vi "load_recipes.vi"(8 "error in (no error)":errorcluster, 11 "recipe":T2) -> (0 "error out":errorcluster, 2 "transition []":string, 3 "recipe []":T1[](array[typedef]))   [LabVIEW 2015, in "lv-recipe-machine.lvlib" / "example_01.lvlib"]
uses:
  example_01.lvlib
  _controls/recipes.ctl
  public/_controls/recipe_step.ctl
  _controls/steps_actions.ctl
  lv-recipe-machine.lvlib
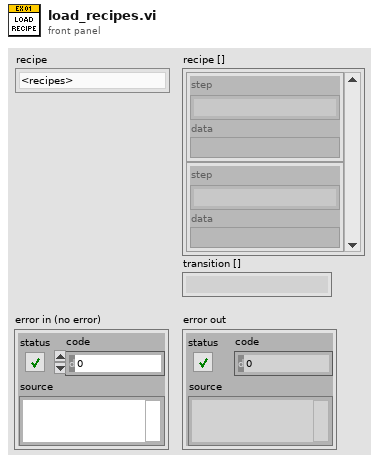
[diagram p1: front panel]
types:
  T1 = typedef "lv-recipe-machine.lvlib/recipe_step.ctl" = cluster{"step":string, "data":variant}
  T2 = typedef "lv-recipe-machine.lvlib/example_01.lvlib/recipes.ctl" = enum16{"<recipes>", "wait_random", "random_wait", "count", "comparison", "launch", "<null>"}
  T3 = typedef "lv-recipe-machine.lvlib/example_01.lvlib/steps_actions.ctl" = enum16{"<steps_actions>", "manual_random", "manual_comparison", "manual_wait", "auto_random", "auto_wait", "criteria_initialize", "criteria_count", "criteria_comparison", "transition_simple", "transition_count", "transition_comparison", "launch_wait", "<null>"}
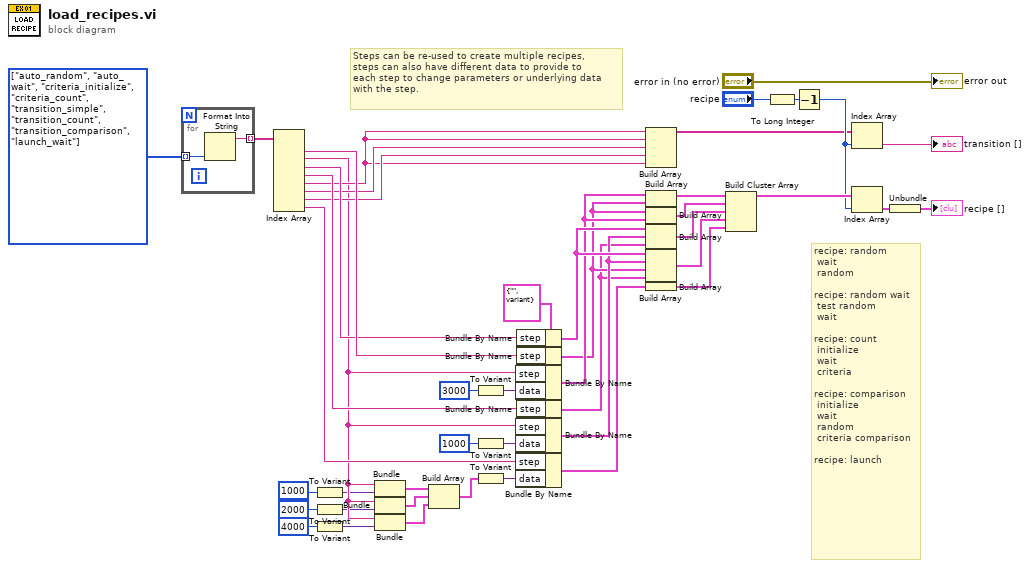
[diagram p0: block diagram]
diagram:
  w31 = T3[] [enum."auto_random", enum."auto_wait", enum."criteria_initialize", enum."criteria_count", enum."transition_simple", enum."transition_count", enum."transition_comparison", enum."launch_wait"] items=["<steps_actions>", "manual_random", "manual_comparison", "manual_wait", "auto_random", "auto_wait", "criteria_initialize", "criteria_count", "criteria_comparison", "transition_simple", "transition_count", "transition_comparison", "launch_wait", "<null>"]
  w17 = T1 {"step"="", "data"=variant} ("lv-recipe-machine.lvlib:recipe_step")
  # "Steps can be re-used to create multiple recipes,\nsteps can also have different data to provide to\neach step to change parameters or underlying data\nwith the step."
  # "recipe: random\n wait\n random \n\nrecipe: random wait\n test random\n wait\n\nrecipe: count\n initialize\n wait\n criteria\n\nrecipe: comparison\n initialize\n wait\n random\n criteria comparison\n\nrecipe: launch"
  n1 = for {
    tunnel: w31 -> [w48] mode=indexing
    tunnel: [w47] -> w30 mode=indexing
    n2 = Format Into String(w48) -> (resulting string=w47:string)  [unwired: 3 in, 1 out]
  }
  n3 = Index Array(array=w30) -> (element #1=w29:string, element #2=w10:string, element #3=w28:string, element #4=w27:string, element #5=w13:string, element #6=w19:string, element #7=w18:string, element #8=w16:string)  [unwired: 8 in]
  n4 = To Variant(anything=1000) -> (Variant=w4:variant)
  n5 = To Variant(anything=2000) -> (Variant=w5:variant)
  n6 = To Variant(anything=4000) -> (Variant=w6:variant)
  n7 = Bundle(w10, "Variant"=w4) -> (w9:cluster{string, "Variant":variant})  [unwired: 1 in]
  n8 = Bundle(w10, "Variant"=w5) -> (w8:cluster{string, "Variant":variant})  [unwired: 1 in]
  n9 = Bundle(w10, "Variant"=w6) -> (w7:cluster{string, "Variant":variant})  [unwired: 1 in]
  n10 = Build Array(w9, w8, w7) -> (w11:cluster{string, "Variant":variant}[])
  n11 = To Variant(anything=3000) -> (Variant=w45:variant)
  n12 = To Variant(anything=1000) -> (Variant=w34:variant)
  n13 = To Variant(anything=w11) -> (Variant=w12:variant)
  n14 = Bundle By Name(cluster=w17, "step"=w10, "data"=w45) -> (w22:T1)
  n15 = Bundle By Name(cluster=w17, "step"=w10, "data"=w34) -> (w23:T1)
  n16 = Bundle By Name(cluster=w17, "step"=w16, "data"=w12) -> (w15:T1)
  n17 = Bundle By Name(cluster=w17, "step"=w28) -> (w25:T1)
  n18 = Bundle By Name(cluster=w17, "step"=w29) -> (w21:T1)
  n19 = Bundle By Name(cluster=w17, "step"=w27) -> (w20:T1)
  n20 = Build Array(w13, w13, w19, w18, w13) -> (w26:string[])
  n21 = Build Array(w22, w21) -> (w36:T1[])
  n22 = Build Array(w21, w22) -> (w35:T1[])
  n23 = Build Array(w25, w23, w20) -> (w32:T1[])
  n24 = Build Array(w25, w23, w21, w20) -> (w24:T1[])
  n25 = Build Array(w15) -> (w14:T1[])
  n26 = Build Cluster Array(w36, w35, w32, w24, w14) -> (w44:cluster{T1[]}[])
  n27 = To Long Integer(number="recipe") -> (32bit integer=w41:i32)
  n28 = Decrement(x=w41) -> (x-1=w38:i32)
  n29 = Index Array(array=w26, index=w38) -> (element=→"transition []":string)
  n30 = Index Array(array=w44, index=w38) -> (element=w40:cluster{T1[]})
  n31 = Unbundle(w40) -> (→"recipe []":T1[])
  "error out" <- "error in (no error)"
